vi "hist.vi"(8 "#clock cycles":u32=10000, 9 "#bins":u32=10, 10 "counter timetag list":u32[](array[numeric])) -> (3 "histogram":i32[](array[numeric]))   [LabVIEW 2014]
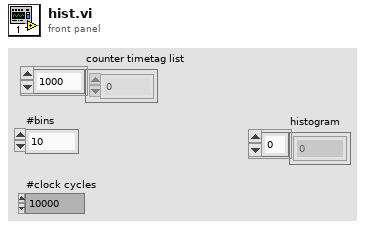
[diagram p1: front panel]
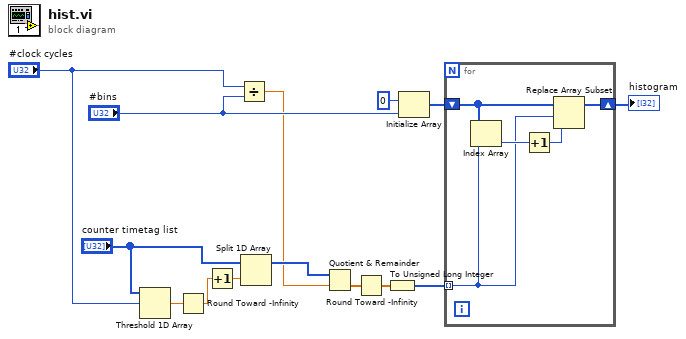
[diagram p0: block diagram]
diagram:
  n1 = Threshold 1D Array(2:"#clock cycles", 3:"counter timetag list") -> (0:w14:dbl)  [unwired: 1 in]
  n2 = Round Toward -Infinity(1:w14) -> (0:w1:dbl)
  n3 = Increment(x=w1) -> (x+1=w2:dbl)
  n4 = Divide(x="#clock cycles", y="#bins") -> (x/y=w4:dbl)
  n5 = Split 1D Array(array="counter timetag list", index=w2) -> (first subarray=w10:u32[])  [unwired: 1 out]
  n6 = Quotient & Remainder(x=w10, y=w4) -> (floor(x/y)=w11:dbl[])  [unwired: 1 out]
  n7 = Round Toward -Infinity(1:w11) -> (0:w12:dbl[])
  n8 = To Unsigned Long Integer(number=w12) -> (unsigned 32bit integer=w9:u32[])
  n9 = Initialize Array(u32 0 ("element"), "#bins") -> (w8:u32[])
  n10 = for {
    shift-right: [w19] -> w3
    shift-left: w8 -> [w18]
    tunnel: w9 -> [w15] mode=indexing
    n11 = Index Array(array=w18, index=w15) -> (element=w17:u32)
    n12 = Increment(x=w17) -> (x+1=w16:u32)
    n13 = Replace Array Subset(array=w18, new element=w16, index=w15) -> (w19:u32[])
  }
  "histogram" <- w3
